vi "Stop Core.vi"(10 "final error code":i32, 11 "Auto UI in":refnum<class "Auto UI.lvclass">) -> (3 "Auto UI out":refnum<class "Auto UI.lvclass">)   [LabVIEW 2023, in "GUI.lvlib" / "Auto UI.lvlib" / "Auto UI.lvclass"]
doc: "(<B>Filename</B>: Actor Framework.lvlib:Actor.lvclass:Stop Core.vi)\n\nDefines what the actor does before it stops. Use the <B>final error code</B> input to determine whether the actor shut down in response to an error.\n\nBy default, this method passes the Stop message along to all auto-stop nested actors. A descendant class may override this method to define additional behavior, such as shutting down any processes the actor initiated in its override of the Actor Core method."
uses:
  Auto UI.lvclass
  Reused Code/Subpanels Actor/subpanels/subpanel/subpanel (abstract).lvclass
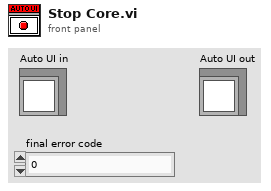
[diagram p1: front panel]
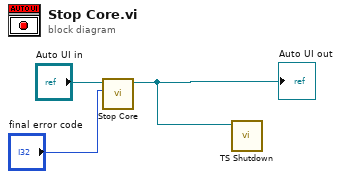
[diagram p0: block diagram]
diagram:
  n1 = call-parent "Stop Core.vi"("final error code"="final error code", "Actor in"="Auto UI in") -> ("Actor out"=w1:refnum<class "Auto UI.lvclass">)  [unwired: 9 in]
  "Auto UI out" <- w1
  n2 = call "TS Shutdown.vi"("Auto UI in"=w1) -> ()  [unwired: 9 in, 2 out]
